vi "PH_Sixpack.calc Axis Acticity.vi"(0 "Endswitch?":bool, 1 "Sign change":bool, 2 "Motor Type":T1, 4 "CurrentActivity":T2, 5 "Input in":T4) -> (16 "Axis Activity":T3, 18 "Running":bool)   [LabVIEW 2014, in "PH_Sixpack.lvlib"]
doc: "This VI calculates the activity of a sixpack axis."
uses:
  PH_Sixpack.lvlib
  PH_Sixpack.Input.ctl
  PH_Stepmotor_BaseClass/PH_Stepmotor_BaseClass.Axis Activity.ctl
  instr.lib/SixPack/PackDLL/Activity.ctl
  PH_Stepmotor_BaseClass/PH_Stepmotor_BaseClass.Motor Type.ctl
  PH_Stepmotor_BaseClass/PH_Stepmotor_BaseClass.lvlib
  instr.lib/SixPack/Sixpack - Driver.lvlib
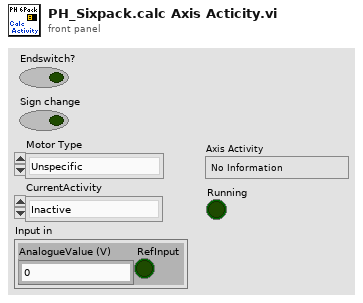
[diagram p1: front panel]
types:
  T1 = typedef "PH_Stepmotor_BaseClass.lvlib/PH_Stepmotor_BaseClass.Motor Type.ctl" = enum16{"Unspecific", "OWIS 49.120.2633", "OWIS 49.060.1033", "OWIS 43.040.2558", "Diamond Motion 2200 series", "OWIS 49.120.266B.MV6", "Calorimeter", "Linear Stage 1", "MICOS VT-80", "MICOS VT-80 S", "Standa Rotstage nt0.95A", "PUF RA 320.200", "PUF RA 800.200", "PUF RA 800.400", "PUF RA 400.50", "1324.nn.800.50", "1324.n9c.800.50", "1324.nn.320.200", "1324.nn.400.200", "1324.nn.800.200", "1324.nn.400.50", "1324.8c9c.800.50", "1324.8c9c.400.200"}
  T2 = typedef "Sixpack - Driver.lvlib/Activity.ctl" = enum16{"Inactive", "Ramp", "PI-Controller", "Rotation", "ReferenceSearch", "Reference Search", "MechanicalReference"}
  T3 = typedef "PH_Stepmotor_BaseClass.lvlib/PH_Stepmotor_BaseClass.Axis Activity.ctl" = enum16{"No Information", "stopped", "running", "Failure", "Alarm", "stopped at backward ES", "stopped at foreward ES"}
  T4 = typedef "PH_Sixpack.lvlib/PH_Sixpack.Input.ctl" = cluster{"AnalogueValue (V)":dbl, "RefInput":bool}
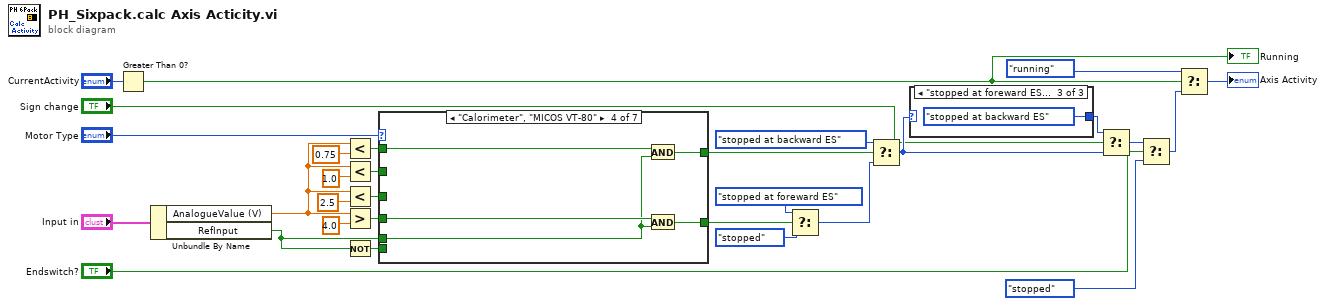
[diagram p0: block diagram]
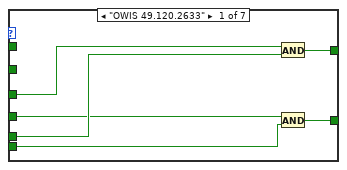
[diagram p2: hidden frame]
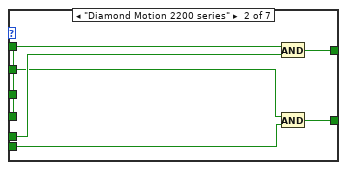
[diagram p3: hidden frame]
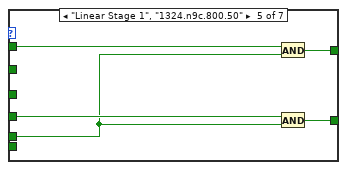
[diagram p5: hidden frame]
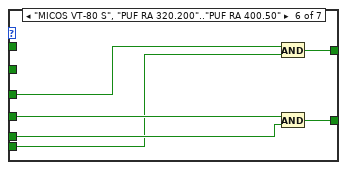
[diagram p6: hidden frame]
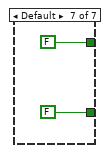
[diagram p7: hidden frame]
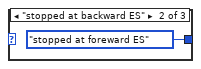
[diagram p9: hidden frame]
diagram:
  n1 = Greater Than 0?(x="CurrentActivity") -> (x > 0?=w10:bool)
  "Running" <- w10
  n2 = Unbundle By Name("Input in") -> ("AnalogueValue (V)"=w6:dbl, "RefInput"=w7:bool)
  n3 = Less?(x=w6, y=0.75) -> (x < y?=w25:bool)
  n4 = Less?(x=w6, y=1.0) -> (x < y?=w24:bool)
  n5 = Less?(x=w6, y=2.5) -> (x < y?=w4:bool)
  n6 = Greater?(x=w6, y=4.0) -> (0:w23:bool)
  n7 = Not(x=w7) -> (.not. x?=w22:bool)
  n8 = case shown="\"Calorimeter\", \"MICOS VT-80\"" "Motor Type" {
    tunnel: w7 -> [w36 w41 _ w45 w52 w59 _]
    tunnel: w25 -> [_ _ _ w49 w54 _ _]
    tunnel: w24 -> [_ w40 w43 _ _ _ _]
    tunnel: w23 -> [w35 w42 w44 w48 w53 w60 _]
    tunnel: w22 -> [w34 w39 _ _ _ w58 _]
    tunnel: [w33 w38 w44 w47 w51 w57 FALSE] -> w26
    tunnel: [w32 w37 w43 w46 w50 w56 FALSE] -> w27
    tunnel: w4 -> [w31 _ _ _ _ w55 _]
    frame "OWIS 49.120.2633" {
      n9 = And(x=w31, y=w36) -> (x .and. y?=w33:bool)
      n10 = And(x=w35, y=w34) -> (x .and. y?=w32:bool)
    }
    frame "Diamond Motion 2200 series" {
      n11 = And(x=w42, y=w41) -> (x .and. y?=w38:bool)
      n12 = And(x=w40, y=w39) -> (x .and. y?=w37:bool)
    }
    frame "OWIS 49.120.266B.MV6" {
    }
    frame "Calorimeter", "MICOS VT-80" {
      n13 = And(x=w49, y=w45) -> (x .and. y?=w47:bool)
      n14 = And(x=w48, y=w45) -> (x .and. y?=w46:bool)
    }
    frame "Linear Stage 1", "1324.n9c.800.50" {
      n15 = And(x=w54, y=w52) -> (x .and. y?=w51:bool)
      n16 = And(x=w53, y=w52) -> (x .and. y?=w50:bool)
    }
    frame "MICOS VT-80 S", "PUF RA 320.200".."PUF RA 400.50" {
      n17 = And(x=w55, y=w58) -> (x .and. y?=w57:bool)
      n18 = And(x=w60, y=w59) -> (x .and. y?=w56:bool)
    }
    frame Default {
    }
  }
  n19 = Select(t=PH_Stepmotor_BaseClass.Axis_Activity."stopped at foreward ES" ("Axis Activity"), s=w27, f=PH_Stepmotor_BaseClass.Axis_Activity."stopped" ("Axis Activity")) -> (s? t:f=w19:T3)
  n20 = Select(t=PH_Stepmotor_BaseClass.Axis_Activity."stopped at backward ES" ("Axis Activity"), s=w26, f=w19) -> (s? t:f=w16:T3)
  n21 = case shown="\"stopped at foreward ES\"" w16 {
    selector: w16 -> [w63 _ _]
    tunnel: [w63 PH_Stepmotor_BaseClass.Axis_Activity."stopped at foreward ES" ("Axis Activity") PH_Stepmotor_BaseClass.Axis_Activity."stopped at backward ES" ("Axis Activity")] -> w17
    frame Default {
    }
    frame "stopped at backward ES" {
    }
    frame "stopped at foreward ES" {
    }
  }
  n22 = Select(t=w17, s="Sign change", f=w16) -> (s? t:f=w28:T3)
  n23 = Select(t=w28, s="Endswitch?", f=PH_Stepmotor_BaseClass.Axis_Activity."stopped" ("Axis Activity")) -> (s? t:f=w29:T3)
  n24 = Select(t=PH_Stepmotor_BaseClass.Axis_Activity."running" ("Axis Activity"), s=w10, f=w29) -> (s? t:f=→"Axis Activity":T3)
